vi "assemble.vi"(8 "error in (no error)":errorcluster, 11 "ChairWithTableAttached in":refnum<class "ChairWithTableAttached.lvclass">) -> (0 "error out":errorcluster, 2 "String":string, 3 "ChairWithTableAttached out":refnum<class "ChairWithTableAttached.lvclass">)   [LabVIEW 2021, in "ChairWithTableAttached.lvclass"]
uses:
  ChairWithTableAttached.lvclass
  ChairWithTableAttached.lvclass/ChairWithTableAttached.ctl
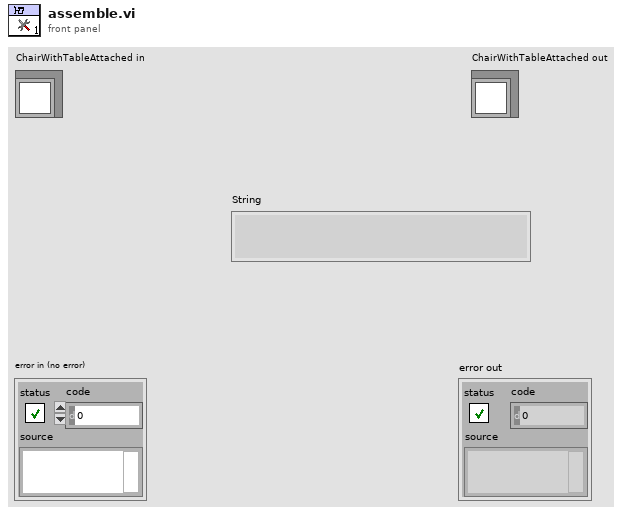
[diagram p1: front panel]
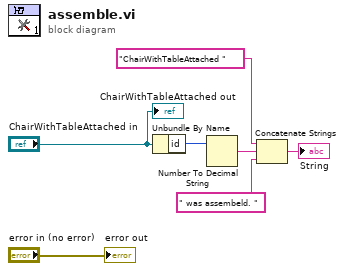
[diagram p0: block diagram]
diagram:
  n1 = Unbundle By Name("ChairWithTableAttached in") -> ("id"=w6:u32)
  n2 = Number To Decimal String(number=w6) -> (decimal integer string=w7:string)  [unwired: 1 in]
  n3 = Concatenate Strings("ChairWithTableAttached ", w7, " was assembeld. ") -> (→"String":string)
  "error out" <- "error in (no error)"
  "ChairWithTableAttached out" <- "ChairWithTableAttached in"
